vi "Reset Assertions.vi"(10 "Run Queue":set{string}(c389), 11 "Result Model In":refnum<class "Result Model.lvclass">) -> (3 "Result Model Out":refnum<class "Result Model.lvclass">)   [LabVIEW 2020, in "Result Model.lvclass"]
uses:
  Result Model.lvclass
  Result Model.lvclass/Result Model.ctl
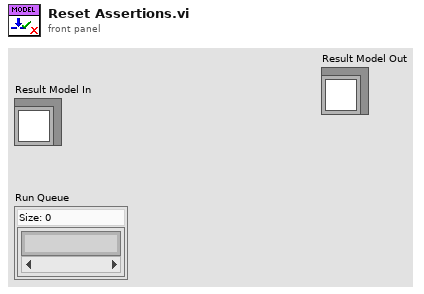
[diagram p1: front panel]
types:
  T1 = typedef "Result.lvlib/Type.ctl" = enum16{"Test Case", "Test Suite", "Test Run", "Pass", "Fail", "Skip", "Pass if", "Fail if", "Pass if Error", "Fail if Error", "Pass if Equal", "Fail if Equal"}
  T2 = typedef "Result.lvlib/Status.ctl" = enum16{"", "Passed", "Failed", "Error", "Skipped", "Setup Error", "Broken", "Teardown Error"}
  T3 = map{string, cluster{"Result Type":T1, "Status":T2, "Message":string, "Description":string}[]}
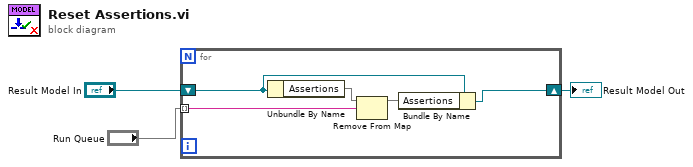
[diagram p0: block diagram]
diagram:
  n1 = for {
    tunnel: "Run Queue" -> [w8] mode=indexing
    shift-right: [w4] -> w1
    shift-left: "Result Model In" -> [w5]
    n2 = Unbundle By Name(w5) -> ("Assertions"=w7:T3)
    n3 = Remove From Map(10:w8, 11:w7) -> (3:w6:T3)  [unwired: 2 out]
    n4 = Bundle By Name(cluster=w5, "Assertions"=w6) -> (w4:refnum<class "Result Model.lvclass">)
  }
  "Result Model Out" <- w1
